vi "Frames.Lookup.Size.Get.vi"(6 "Type":T1=enum."DTC Control", 8 "error in (no error)":errorcluster, 10 "ID":u32, 11 "Frames Lookup":variant) -> (0 "error out":errorcluster, 2 "ByteLength":u16, 3 "found":bool)   [LabVIEW 2019, in "Diagnostics Addon Engine.lvlib"]
uses:
  Diagnostics Addon Engine.lvlib
  Shared/Types/Type.ctl
  Shared/Types/Frame.Lookup.Info.ctl
  Shared/Diagnostics Addon Shared.lvlib
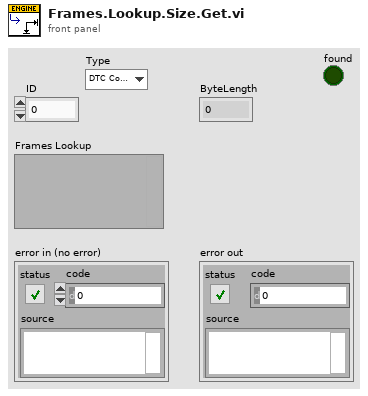
[diagram p1: front panel]
types:
  T1 = typedef "Diagnostics Addon Shared.lvlib/Type.ctl" = enum16{"DID", "CDID", "PID", "CPID", "Read Memory", "Write Memory", "DTC Control", "IO Cmd", "IO Resp", "Routine Start Cmd", "Routine Start Resp", "Routine Request Cmd", "Routine Request Resp", "Routine Stop Cmd", "Routine Stop Resp", "UserDefined Cmd", "UserDefined Rsp"}
  T2 = typedef "Diagnostics Addon Shared.lvlib/Frame.Lookup.Info.ctl" = cluster{"Offset":i32, "Length":i32, "ByteLength":u16}
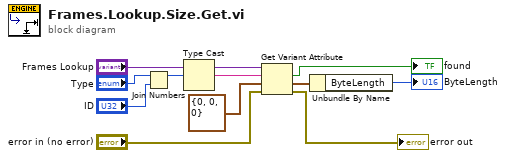
[diagram p0: block diagram]
diagram:
  n1 = Join Numbers(hi="Type", lo="ID") -> ((hi.lo)=w4:u64)
  n2 = Type Cast(x=w4) -> (*(type *) &x=w5:string)  [unwired: 1 in]
  n3 = Get Variant Attribute(Variant="Frames Lookup", name=w5, default value (empty Variant)=T2 {"Offset"=0, "Length"=0, "ByteLength"=0} ("cluster"), error in="error in (no error)") -> (found=→"found":bool, value=w7:T2, error out=→"error out":errorcluster)  [unwired: 1 out]
  n4 = Unbundle By Name(w7) -> ("ByteLength"=→"ByteLength":u16)
